vi "test Logging Loopback.vi"(8 "error in":errorcluster, 11 "TestCase in":refnum<class "Logging Loopback.lvclass">) -> (0 "error out":errorcluster, 3 "TestCase out":refnum<class "Logging Loopback.lvclass">)   [LabVIEW 2020, in "Logging Loopback.lvclass"]
uses:
  Logging Loopback.lvclass
  <vilib>/addons/_JKI Toolkits/VI Tester/TestCase.llb/TestCase.lvclass
  <vilib>/NI VeriStand/Execution/Workspace/NI_VS Workspace ExecutionAPI.lvlib
  niveristand-custom-device-testing-tools/VeriStandTestUtilities/VeriStandTestUtilities.lvlib
  <vilib>/NI VeriStand/Execution/Workspace/NI VeriStand - Set Multiple Channel Values.vi
  <vilib>/NI VeriStand/Execution/Workspace/NI VeriStand - Get Multiple Channel Values.vi
  deffbcbf-56d6-44bc-a2e8-818e5af24b3f.vi
  <vilib>/NI VeriStand/Execution/Workspace/NI VeriStand - Get Single Channel Value.vi
  6b2bfa70-eeaf-4af2-80f2-6a86f8a7f598.vi
  <vilib>/NI VeriStand/Execution/Workspace/NI VeriStand - Set Single Channel Value.vi
  8c6fca9a-303d-43f5-9dd5-93be59ae7e12.vi
  8e29fdbb-99f4-44e6-93c0-7b36a3c9813a.vi
  f1b300ac-3edd-4135-92f3-1091e6e89550.vi
  <vilib>/numeric/Random Number (Range) U64.vi
  48c03b12-561d-41cc-966c-8db0e8e8288a.vi
  73f23597-aef4-4ff6-a202-43428571e7d8.vi
  14110b57-2ec4-40ff-8532-aa1d9e607739.vi
  11a182cf-1dad-4243-940f-e832a48a190d.vi
  ddb50979-a497-467d-9150-38dd6115816f.vi
  db7b1ca4-f33a-45a5-961e-f51998a9de3e.vi
  C:/dev/niveristand-custom-device-testing-tools/VeriStandTestCase/VeriStandTestCase.lvclass
  C:/Program Files (x86)/National Instruments/LabVIEW 2020/vi.lib/addons/_JKI Toolkits/VI Tester/TestCase.llb/TestCase.lvclass
  C:/dev/niveristand-ballard-milStd1553-custom-device/Source/Custom Device Support/Tests/System/Logging Loopback/Logging Loopback.lvclass
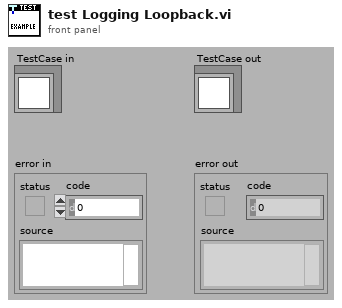
[diagram p1: front panel]
types:
  T1 = typedef "NI_VS Workspace ExecutionAPI.lvlib/WorkspaceAPI.ctl" = refnum<k24>
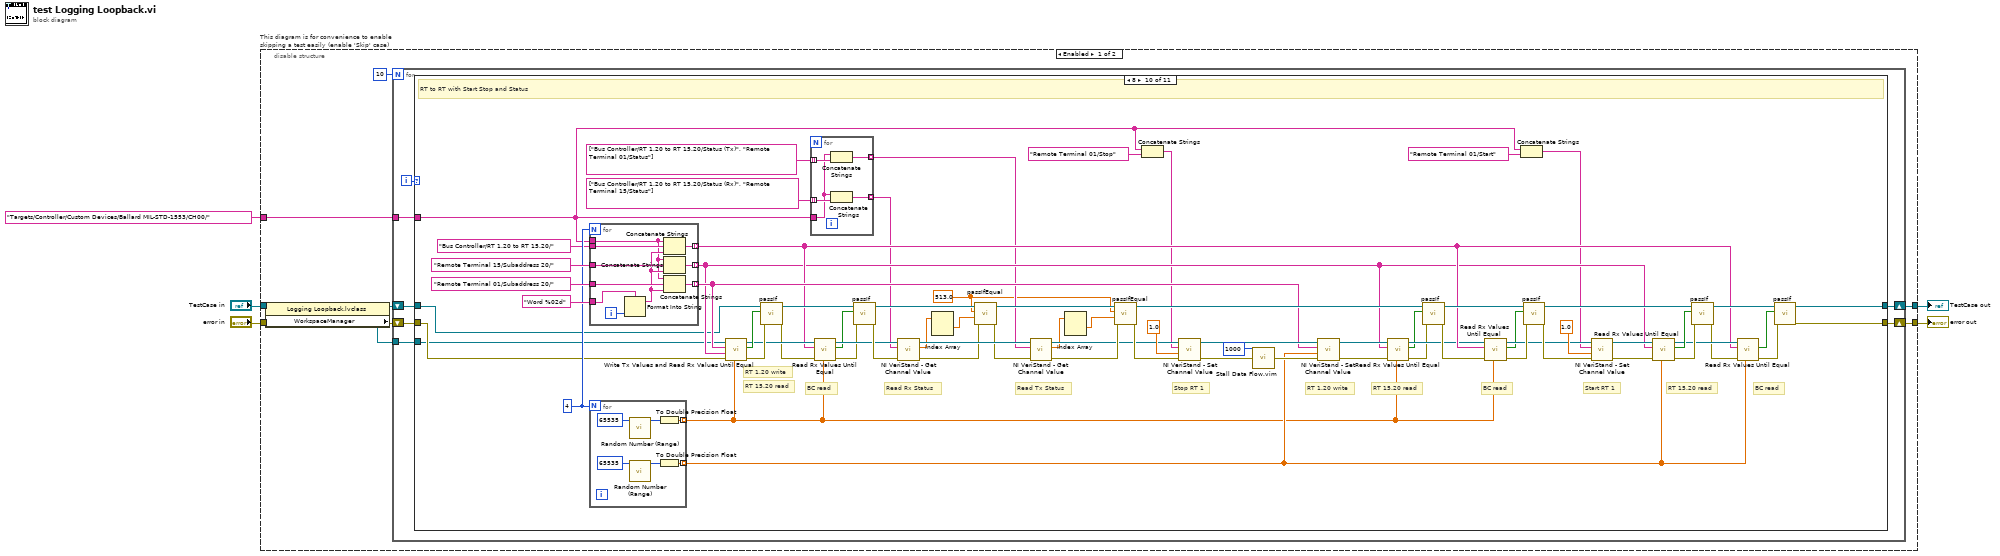
[diagram p0: block diagram]
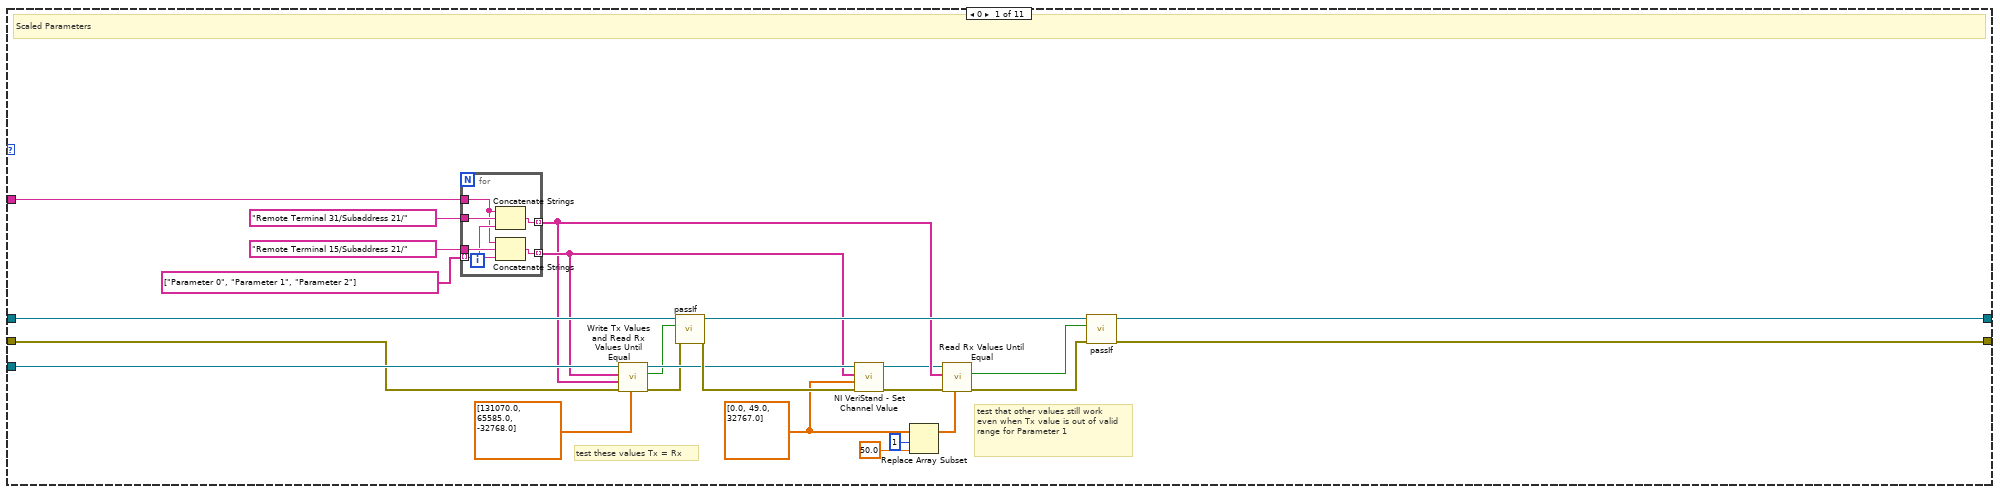
[diagram p2: hidden frame]
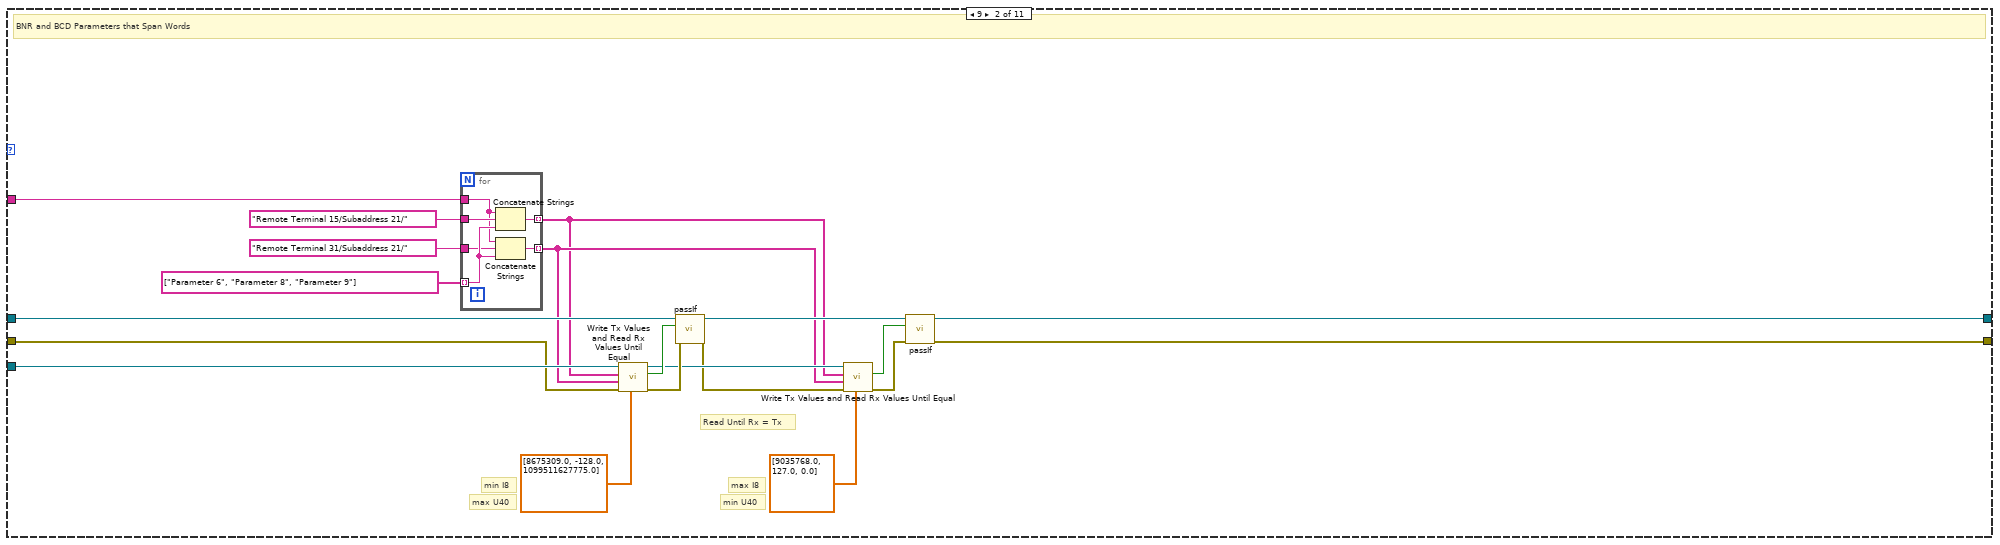
[diagram p3: hidden frame]
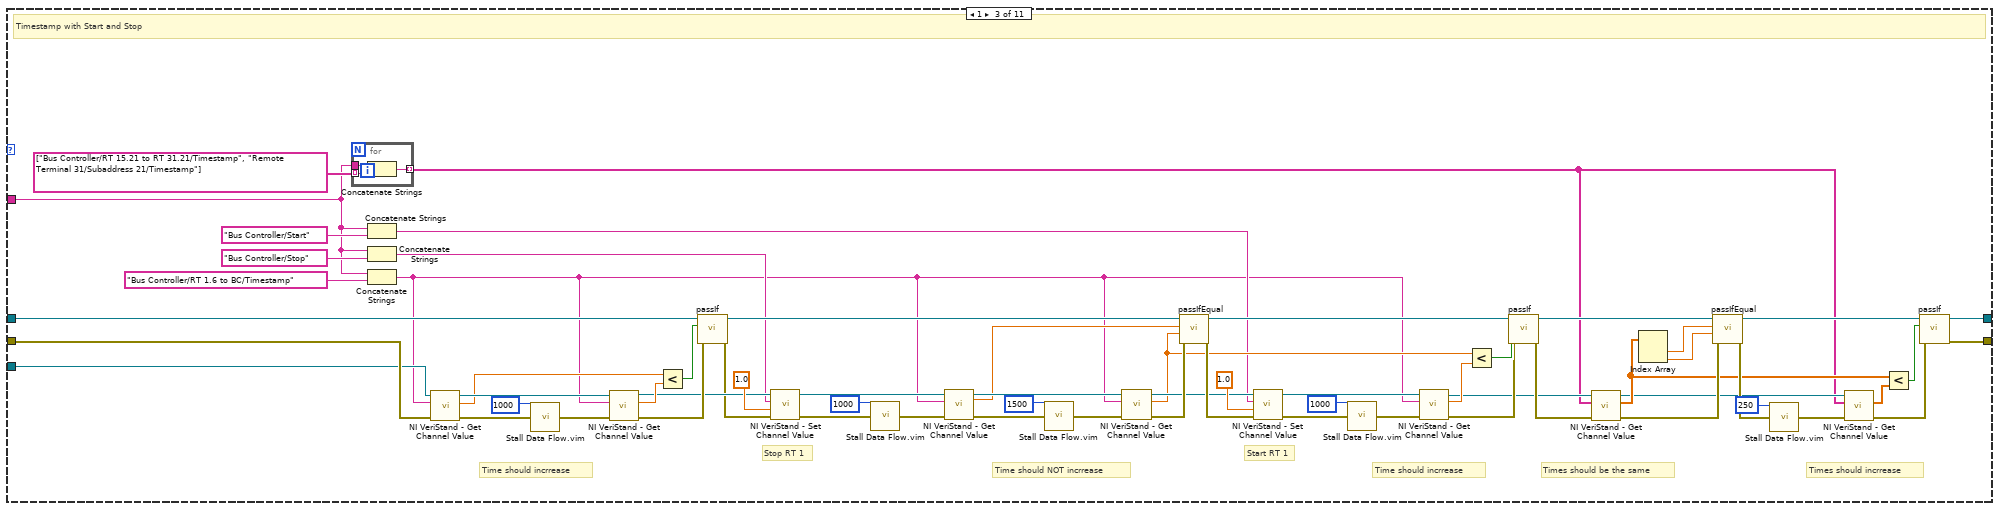
[diagram p4: hidden frame]
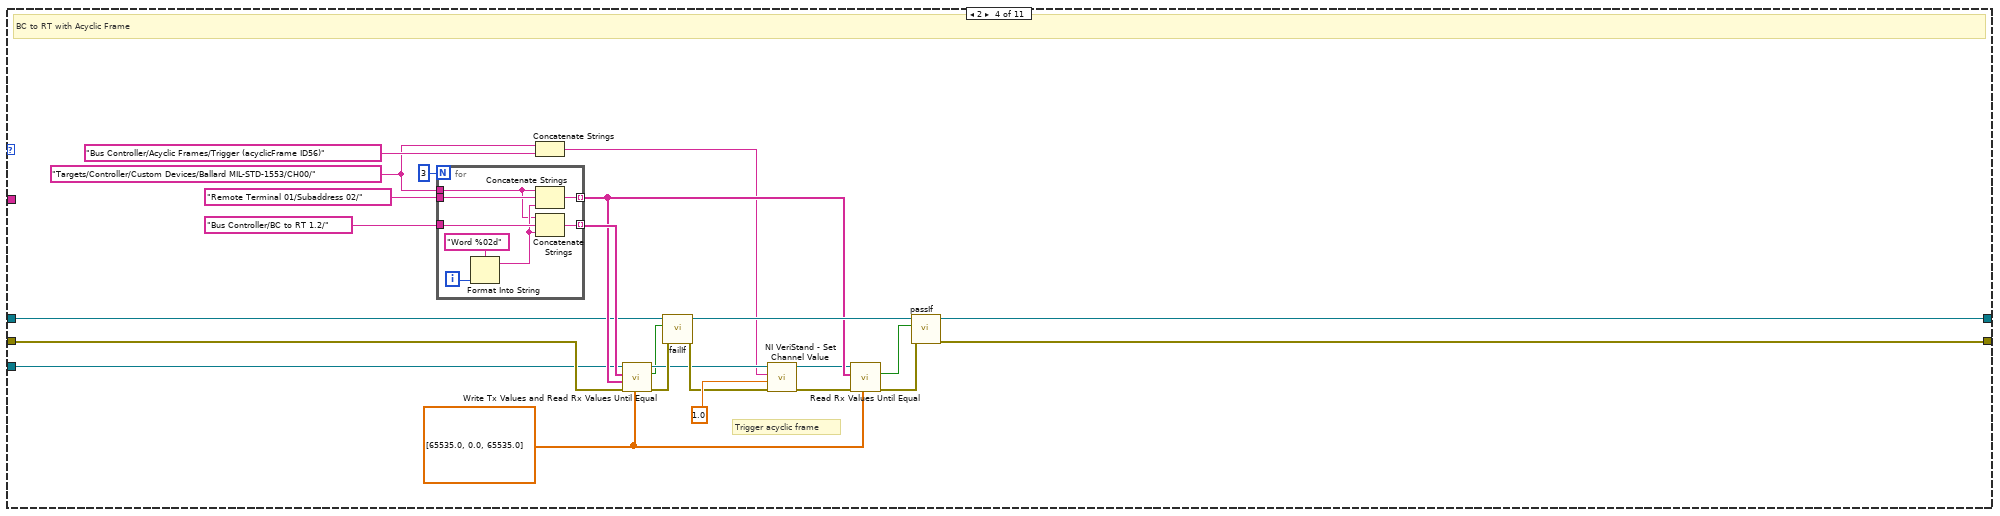
[diagram p5: hidden frame]
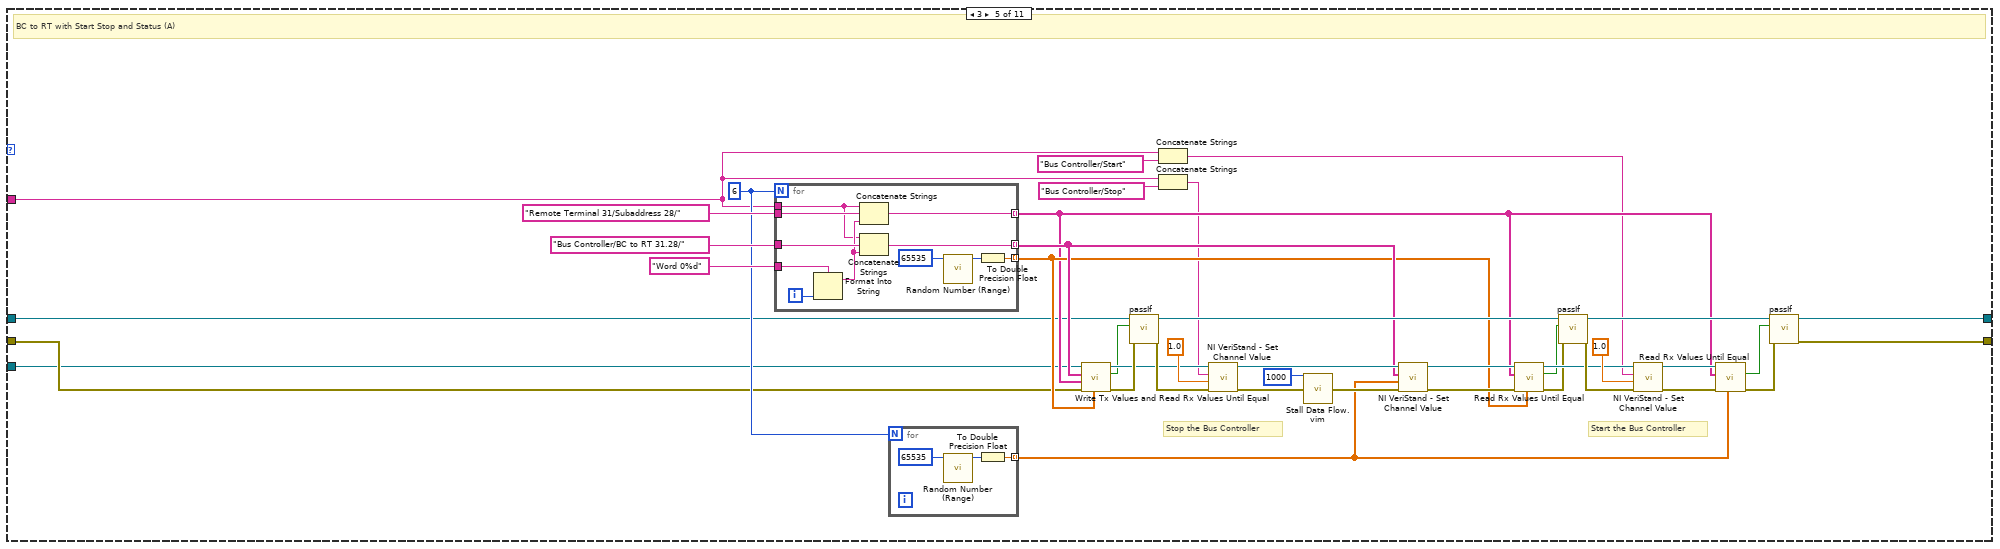
[diagram p6: hidden frame]
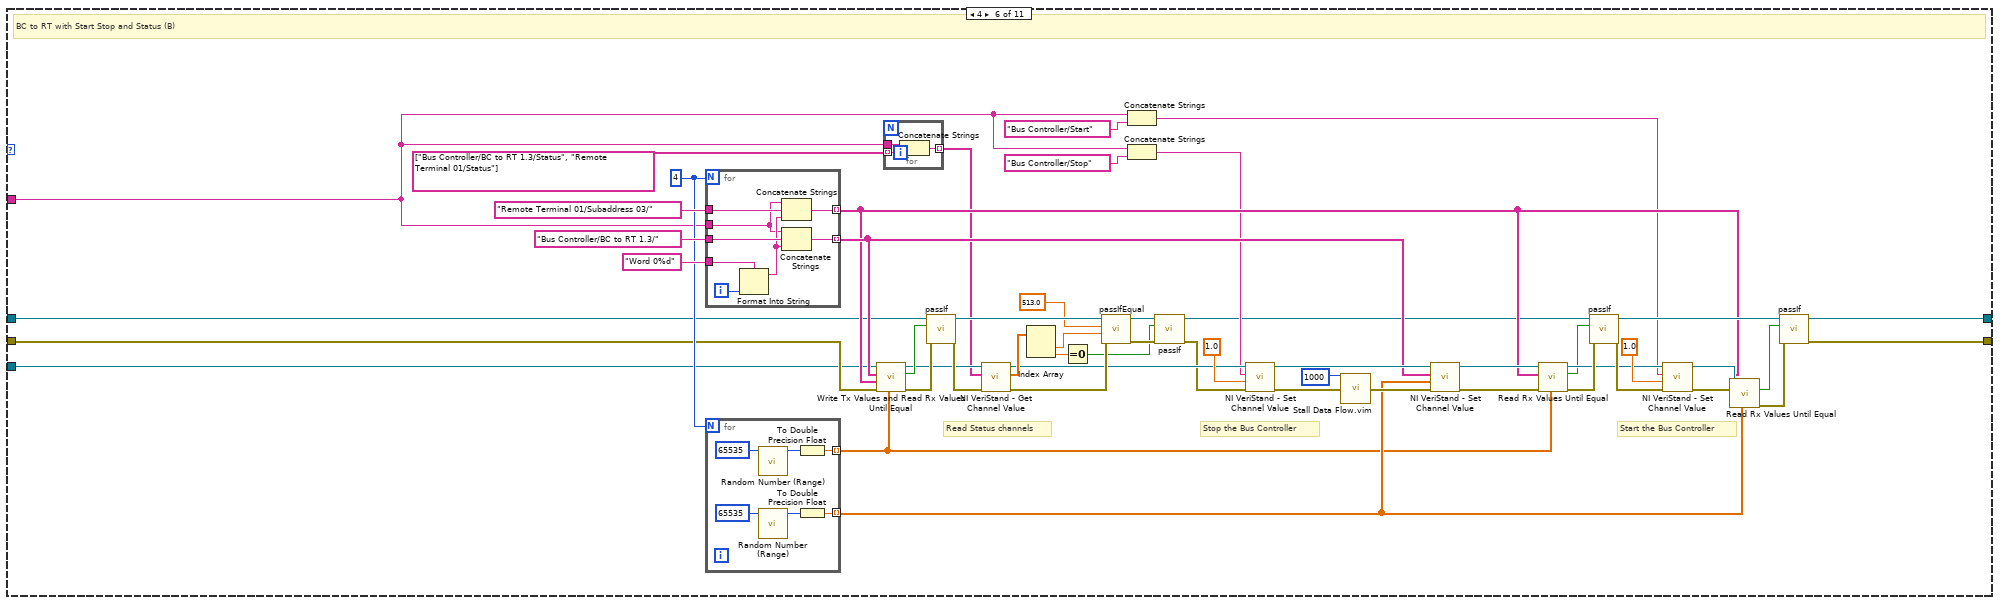
[diagram p7: hidden frame]
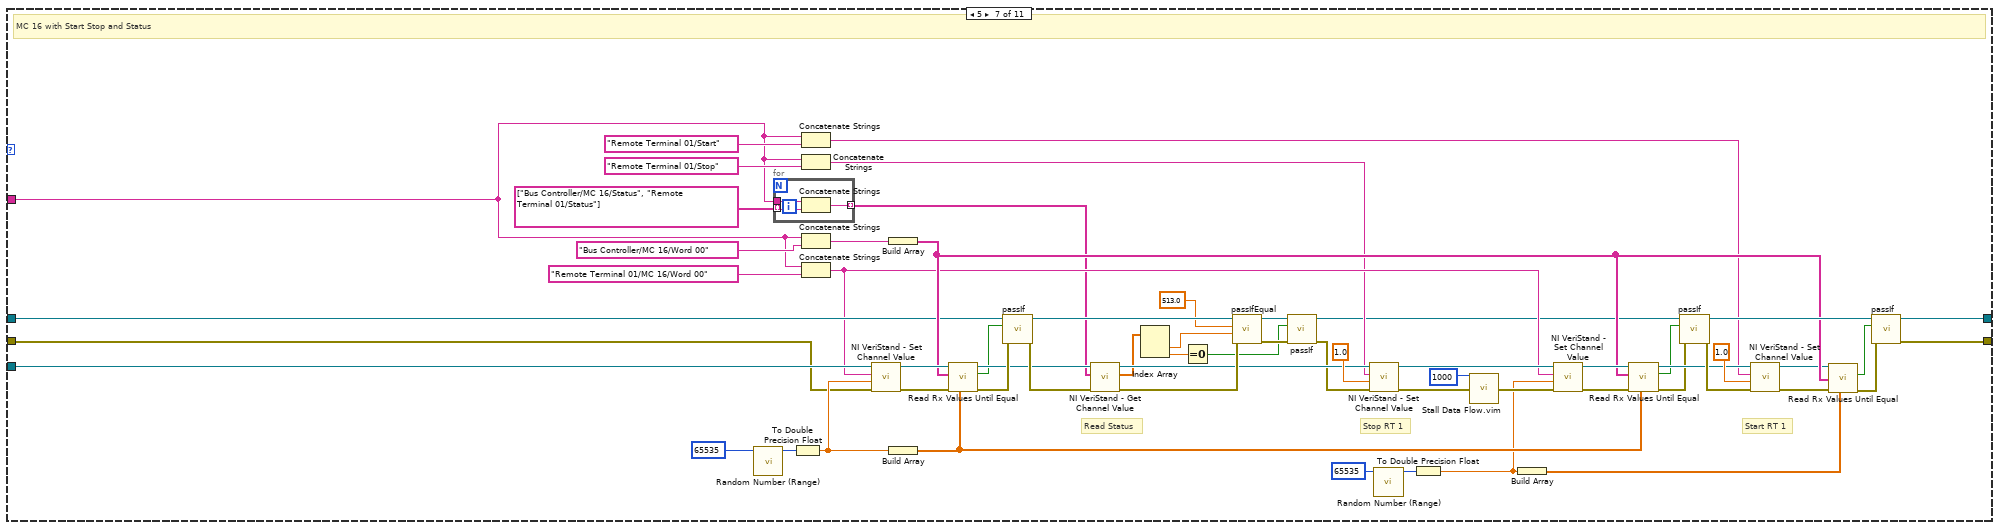
[diagram p8: hidden frame]
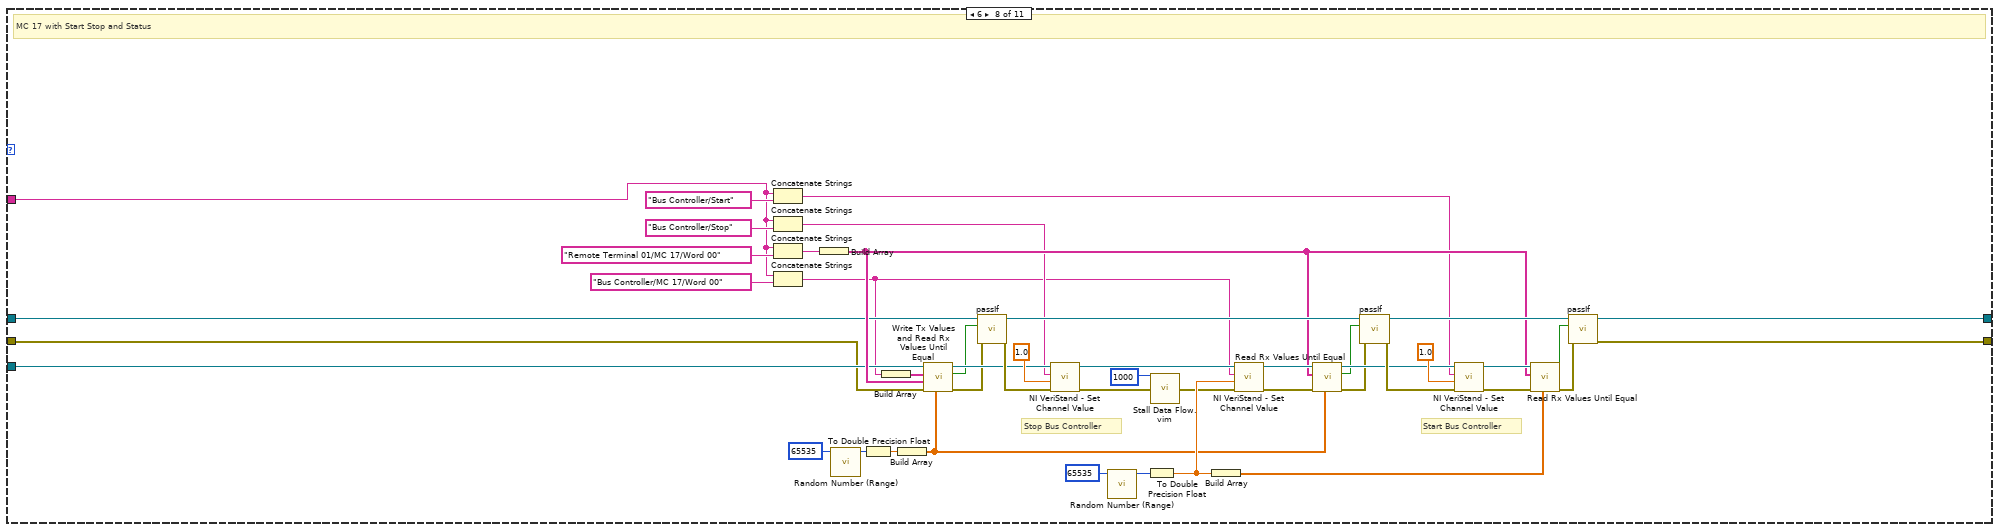
[diagram p9: hidden frame]
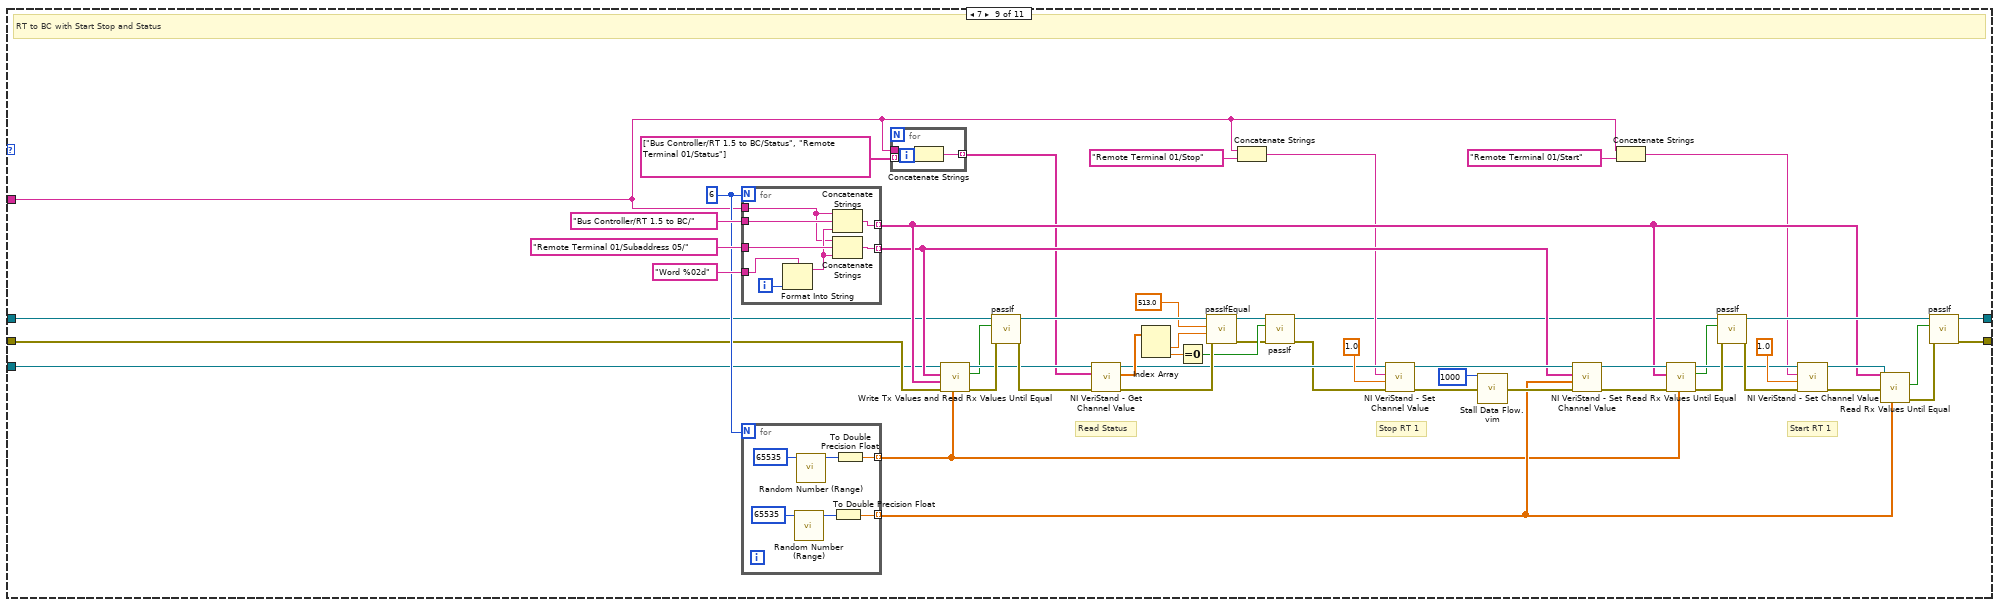
[diagram p10: hidden frame]
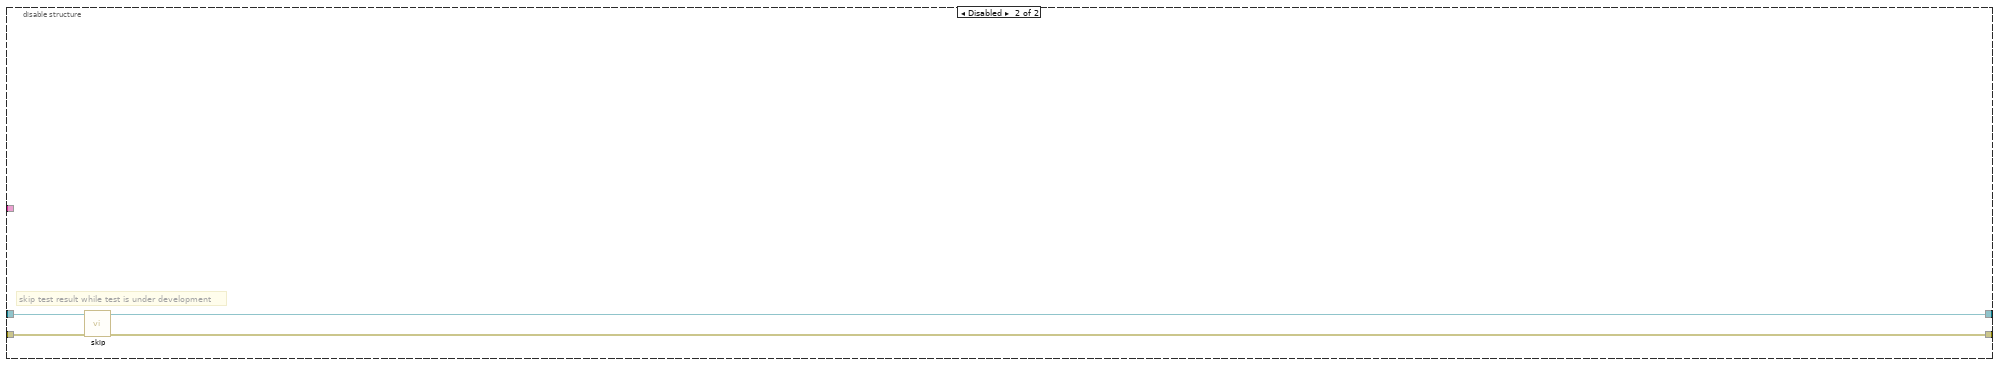
[diagram p12: hidden frame]
diagram:
  n1 = disable-structure "This diagram is for convenience to enable skipping a test easily (enable 'Skip' case)" shown="Enabled" {
    disable-tunnel: "TestCase in" -> [w13 w580]
    disable-tunnel: [w11 w578] -> w2
    disable-tunnel: [w10 w579] -> w4
    disable-tunnel: "error in" -> [w12 w577]
    disable-tunnel: "Targets/Controller/Custom Devices/Ballard MIL-STD-1553/CH00/" ("Channel") -> [w7 _]
    frame Enabled {
      n2 = property class="Logging Loopback.lvclass"(reference=w13, error in=w12) -> (reference out=w14:refnum<class "Logging Loopback.lvclass">, error out=w8:errorcluster, "WorkspaceManager"=w9:T1)
      n3 = for {
        N: 10 -> [_]
        tunnel: w9 -> [w18]
        tunnel: w7 -> [w16]
        shift-right: [w20] -> w11
        shift-left: w14 -> [w21]
        shift-right: [w19] -> w10
        shift-left: w8 -> [w17]
        i -> [w15]
        n4 = case shown="8" w15 {
          tunnel: w21 -> [w46 w72 w85 w149 w177 w243 w323 w375 w429 w483 w576]
          tunnel: [w40 w67 w81 w146 w179 w240 w320 w377 w426 w485 w576] -> w20
          tunnel: [w39 w66 w80 w145 w178 w239 w321 w376 w425 w484 w575] -> w19
          tunnel: w18 -> [w36 w65 w83 w147 w185 w241 w324 w374 w427 w495 _]
          tunnel: w17 -> [w33 w63 w84 w148 w186 w242 w322 w373 w428 w496 w575]
          tunnel: w16 -> [w22 w60 w79 _ w180 w245 w311 w364 w418 w487 _]
          frame 0 {
            w24 = dbl[] [0.0, 49.0, 32767.0] ("appended array")
            # "test that other values still work even when Tx value is out of valid range for Parameter 1"
            # "test these values Tx = Rx"
            # "Scaled Parameters"
            n5 = for {
              tunnel: "Remote Terminal 15/Subaddress 21/" ("Channel") -> [w51]
              tunnel: string[] ["Parameter 0", "Parameter 1", "Parameter 2"] ("Channels") -> [w50] mode=indexing
              tunnel: [w52] -> w31 mode=indexing
              tunnel: "Remote Terminal 31/Subaddress 21/" ("Channel") -> [w49]
              tunnel: [w48] -> w30 mode=indexing
              tunnel: w22 -> [w47]
              n6 = Concatenate Strings(w47, w49, w50) -> (w48:string)
              n7 = Concatenate Strings(w47, w51, w50) -> (w52:string)
            }
            n8 = call "Write Tx Values and Read Rx Values Until Equal.vi"("Tx values"=dbl[] [131070.0, 65585.0, -32768.0] ("appended array"), "error in"=w33, "Rx aliases"=w30, "Tx aliases"=w31, "workspace manager in"=w36) -> ("error out"=w34:errorcluster, "values equal"=w32:bool, "workspace manager out"=w35:T1)  [unwired: 4 in]
            n9 = call-dynamic "passIf.vi"("error in (no error)"=w34, "pass"=w32, "TestCase in"=w46) -> ("error out"=w42:errorcluster, "TestCase out"=w41:refnum<class "Logging Loopback.lvclass">)  [unwired: 7 in]
            n10 = call-poly <vilib>:"NI VeriStand - Set Channel Value.vi"("error in (no error)"=w42, "Values"=w24, "Channels"=w31, "WorkspaceManager in"=w35) -> ("error out"=w29:errorcluster, "WorkspaceManager out"=w28:T1)  [unwired: 6 in]
            n11 = Replace Array Subset(array=w24, new element=50.0 ("x+y"), index=1) -> (w27:dbl[])
            n12 = call "Read Rx Values Until Equal.vi"("expected values"=w27, "error in"=w29, "Rx aliases"=w30, "workspace manager in"=w28) -> ("error out"=w25:errorcluster, "values equal expected"=w26:bool)  [unwired: 5 in, 1 out]
            n13 = call-dynamic "passIf.vi"("error in (no error)"=w25, "pass"=w26, "TestCase in"=w41) -> ("error out"=w39:errorcluster, "TestCase out"=w40:refnum<class "Logging Loopback.lvclass">)  [unwired: 7 in]
          }
          frame 9 {
            # "min U40"
            # "Read Until Rx = Tx"
            # "max I8"
            # "min I8"
            # "max U40"
            # "Read Until Rx = Tx"
            # "BNR and BCD Parameters that Span Words"
            n14 = for {
              tunnel: "Remote Terminal 15/Subaddress 21/" ("Channel") -> [w77]
              tunnel: string[] ["Parameter 6", "Parameter 8", "Parameter 9"] ("Channels") -> [w76] mode=indexing
              tunnel: [w78] -> w56 mode=indexing
              tunnel: "Remote Terminal 31/Subaddress 21/" ("Channel") -> [w75]
              tunnel: [w74] -> w57 mode=indexing
              tunnel: w60 -> [w73]
              n15 = Concatenate Strings(w73, w77, w76) -> (w78:string)
              n16 = Concatenate Strings(w73, w75, w76) -> (w74:string)
            }
            n17 = call "Write Tx Values and Read Rx Values Until Equal.vi"("Tx values"=dbl[] [8675309.0, -128.0, 1099511627775.0] ("appended array"), "error in"=w63, "Rx aliases"=w57, "Tx aliases"=w56, "workspace manager in"=w65) -> ("error out"=w64:errorcluster, "values equal"=w62:bool, "workspace manager out"=w59:T1)  [unwired: 4 in]
            n18 = call-dynamic "passIf.vi"("error in (no error)"=w64, "pass"=w62, "TestCase in"=w72) -> ("error out"=w58:errorcluster, "TestCase out"=w68:refnum<class "Logging Loopback.lvclass">)  [unwired: 7 in]
            n19 = call "Write Tx Values and Read Rx Values Until Equal.vi"("Tx values"=dbl[] [9035768.0, 127.0, 0.0] ("appended array"), "error in"=w58, "Rx aliases"=w57, "Tx aliases"=w56, "workspace manager in"=w59) -> ("error out"=w55:errorcluster, "values equal"=w54:bool)  [unwired: 4 in, 1 out]
            n20 = call-dynamic "passIf.vi"("error in (no error)"=w55, "pass"=w54, "TestCase in"=w68) -> ("error out"=w66:errorcluster, "TestCase out"=w67:refnum<class "Logging Loopback.lvclass">)  [unwired: 7 in]
          }
          frame 1 {
            # "Time should incrrease"
            # "Start RT 1"
            # "Time should NOT incrrease"
            # "Stop RT 1"
            # "Times should incrrease"
            # "Times should be the same"
            # "Time should incrrease"
            # "Timestamp with Start and Stop"
            n21 = for {
              tunnel: string[] ["Bus Controller/RT 15.21 to RT 31.21/Timestamp", "Remote Terminal 31/Subaddress 21/Timestamp"] ("Channels") -> [w144] mode=indexing
              tunnel: w79 -> [w143]
              tunnel: [w142] -> w86 mode=indexing
              n22 = Concatenate Strings(w143, w144) -> (w142:string)
            }
            n23 = Concatenate Strings(w79, "Bus Controller/Start" ("Channel")) -> (w91:string)
            n24 = Concatenate Strings(w79, "Bus Controller/Stop" ("Channel")) -> (w89:string)
            n25 = Concatenate Strings(w79, "Bus Controller/RT 1.6 to BC/Timestamp") -> (w82:string)
            n26 = call-poly <vilib>:"NI VeriStand - Get Channel Value.vi"("error in (no error)"=w84, "Channel"=w82, "WorkspaceManager in"=w83) -> ("error out"=w139:errorcluster, "Value"=w135:dbl, "WorkspaceManager out"=w141:T1)  [unwired: 6 in]
            n27 = call "Stall Data Flow.vim"("value in"=w139, "milliseconds to wait"=u32 1000) -> ("value out"=w140:errorcluster)  [unwired: 1 out]
            n28 = call-poly <vilib>:"NI VeriStand - Get Channel Value.vi"("error in (no error)"=w140, "Channel"=w82, "WorkspaceManager in"=w141) -> ("error out"=w137:errorcluster, "Value"=w134:dbl, "WorkspaceManager out"=w118:T1)  [unwired: 6 in]
            n29 = Less?(x=w135, y=w134) -> (x < y?=w133:bool)
            n30 = call-dynamic "passIf.vi"("error in (no error)"=w137, "pass"=w133, "TestCase in"=w85) -> ("error out"=w117:errorcluster, "TestCase out"=w110:refnum<class "Logging Loopback.lvclass">)  [unwired: 7 in]
            n31 = call-poly <vilib>:"NI VeriStand - Set Channel Value.vi"("error in (no error)"=w117, "Value"=1.0, "Channel"=w89, "WorkspaceManager in"=w118) -> ("error out"=w120:errorcluster, "WorkspaceManager out"=w114:T1)  [unwired: 6 in]
            n32 = call "Stall Data Flow.vim"("value in"=w120, "milliseconds to wait"=u32 1000) -> ("value out"=w113:errorcluster)  [unwired: 1 out]
            n33 = call-poly <vilib>:"NI VeriStand - Get Channel Value.vi"("error in (no error)"=w113, "Channel"=w82, "WorkspaceManager in"=w114) -> ("error out"=w115:errorcluster, "Value"=w109:dbl, "WorkspaceManager out"=w112:T1)  [unwired: 6 in]
            n34 = call "Stall Data Flow.vim"("value in"=w115, "milliseconds to wait"=u32 1500) -> ("value out"=w111:errorcluster)  [unwired: 1 out]
            n35 = call-poly <vilib>:"NI VeriStand - Get Channel Value.vi"("error in (no error)"=w111, "Channel"=w82, "WorkspaceManager in"=w112) -> ("error out"=w108:errorcluster, "Value"=w98:dbl, "WorkspaceManager out"=w102:T1)  [unwired: 6 in]
            n36 = call-dynamic "passIfEqual.vi"("error in (no error)"=w108, "y"=w98, "x"=w109, "TestCase in"=w110) -> ("error out"=w103:errorcluster, "TestCase out"=w97:refnum<class "Logging Loopback.lvclass">)  [unwired: 6 in]
            n37 = call-poly <vilib>:"NI VeriStand - Set Channel Value.vi"("error in (no error)"=w103, "Value"=1.0, "Channel"=w91, "WorkspaceManager in"=w102) -> ("error out"=w105:errorcluster, "WorkspaceManager out"=w107:T1)  [unwired: 6 in]
            n38 = call "Stall Data Flow.vim"("value in"=w105, "milliseconds to wait"=u32 1000) -> ("value out"=w101:errorcluster)  [unwired: 1 out]
            n39 = call-poly <vilib>:"NI VeriStand - Get Channel Value.vi"("error in (no error)"=w101, "Channel"=w82, "WorkspaceManager in"=w107) -> ("error out"=w96:errorcluster, "Value"=w99:dbl, "WorkspaceManager out"=w94:T1)  [unwired: 6 in]
            n40 = Less?(x=w98, y=w99) -> (x < y?=w100:bool)
            n41 = call-dynamic "passIf.vi"("error in (no error)"=w96, "pass"=w100, "TestCase in"=w97) -> ("error out"=w95:errorcluster, "TestCase out"=w93:refnum<class "Logging Loopback.lvclass">)  [unwired: 7 in]
            n42 = call-poly <vilib>:"NI VeriStand - Get Channel Value.vi"("error in (no error)"=w95, "Channels"=w86, "WorkspaceManager in"=w94) -> ("error out"=w136:errorcluster, "Values"=w125:dbl[], "WorkspaceManager out"=w123:T1)  [unwired: 6 in]
            n43 = Index Array(array=w125) -> (element #1=w132:dbl, element #2=w131:dbl)  [unwired: 2 in]
            n44 = call-dynamic "passIfEqual.vi"("error in (no error)"=w136, "y"=w131, "x"=w132, "TestCase in"=w93) -> ("error out"=w130:errorcluster, "TestCase out"=w122:refnum<class "Logging Loopback.lvclass">)  [unwired: 6 in]
            n45 = call "Stall Data Flow.vim"("value in"=w130, "milliseconds to wait"=u32 250) -> ("value out"=w128:errorcluster)  [unwired: 1 out]
            n46 = call-poly <vilib>:"NI VeriStand - Get Channel Value.vi"("error in (no error)"=w128, "Channels"=w86, "WorkspaceManager in"=w123) -> ("error out"=w126:errorcluster, "Values"=w124:dbl[])  [unwired: 6 in, 1 out]
            n47 = Less?(x=w125, y=w124) -> (x < y?=w127:bool)
            n48 = call-dynamic "passIf.vi"("error in (no error)"=w126, "pass"=w127, "TestCase in"=w122) -> ("error out"=w80:errorcluster, "TestCase out"=w81:refnum<class "Logging Loopback.lvclass">)  [unwired: 7 in]
          }
          frame 2 {
            w151 = "Targets/Controller/Custom Devices/Ballard MIL-STD-1553/CH00/" ("Channel")
            w153 = dbl[] [65535.0, 0.0, 65535.0]
            # "Trigger acyclic frame"
            # "BC to RT with Acyclic Frame"
            n49 = for {
              N: 3 -> [_]
              tunnel: "Bus Controller/BC to RT 1.2/" ("Channel") -> [w175]
              tunnel: [w176] -> w162 mode=indexing
              tunnel: "Remote Terminal 01/Subaddress 02/" ("Channel") -> [w174]
              tunnel: [w173] -> w160 mode=indexing
              tunnel: w151 -> [w169]
              i -> [w172]
              n50 = Format Into String(format string="Word %02d", w172) -> (resulting string=w171:string)  [unwired: 2 in, 1 out]
              n51 = Concatenate Strings(w169, w174, w171) -> (w173:string)
              n52 = Concatenate Strings(w169, w175, w171) -> (w176:string)
            }
            n53 = Concatenate Strings(w151, "Bus Controller/Acyclic Frames/Trigger (acyclicFrame ID56)") -> (w150:string)
            n54 = call "Write Tx Values and Read Rx Values Until Equal.vi"("Tx values"=w153, "error in"=w148, "Rx aliases"=w160, "Tx aliases"=w162, "workspace manager in"=w147) -> ("error out"=w161:errorcluster, "values equal"=w154:bool, "workspace manager out"=w158:T1)  [unwired: 4 in]
            n55 = call-dynamic "failIf.vi"("error in (no error)"=w161, "fail"=w154, "TestCase in"=w149) -> ("error out"=w164:errorcluster, "TestCase out"=w163:refnum<class "Logging Loopback.lvclass">)  [unwired: 7 in]
            n56 = call-poly <vilib>:"NI VeriStand - Set Channel Value.vi"("error in (no error)"=w164, "Value"=1.0, "Channel"=w150, "WorkspaceManager in"=w158) -> ("error out"=w155:errorcluster, "WorkspaceManager out"=w156:T1)  [unwired: 6 in]
            n57 = call "Read Rx Values Until Equal.vi"("expected values"=w153, "error in"=w155, "Rx aliases"=w160, "workspace manager in"=w156) -> ("error out"=w157:errorcluster, "values equal expected"=w159:bool)  [unwired: 5 in, 1 out]
            n58 = call-dynamic "passIf.vi"("error in (no error)"=w157, "pass"=w159, "TestCase in"=w163) -> ("error out"=w145:errorcluster, "TestCase out"=w146:refnum<class "Logging Loopback.lvclass">)  [unwired: 7 in]
          }
          frame 3 {
            w202 = 6
            # "Start the Bus Controller"
            # "Stop the Bus Controller"
            # "BC to RT with Start Stop and Status (A)"
            n59 = for {
              N: w202 -> [_]
              tunnel: "Bus Controller/BC to RT 31.28/" ("Channel") -> [w226]
              tunnel: [w227] -> w201 mode=indexing
              tunnel: "Remote Terminal 31/Subaddress 28/" ("Channel") -> [w225]
              tunnel: [w224] -> w190 mode=indexing
              tunnel: "Word 0%d" -> [w222]
              tunnel: [w218] -> w195 mode=indexing
              tunnel: w180 -> [w217]
              i -> [w223]
              n60 = Format Into String(format string=w222, w223) -> (resulting string=w221:string)  [unwired: 2 in, 1 out]
              n61 = Concatenate Strings(w217, w225, w221) -> (w224:string)
              n62 = Concatenate Strings(w217, w226, w221) -> (w227:string)
              n63 = call-poly <vilib>:"Random Number (Range).vi"("upper bound (100)"=u64 65535) -> ("number"=w220:u64)  [unwired: 10 in]
              n64 = To Double Precision Float(number=w220) -> (double precision float=w218:dbl)
            }
            n65 = for {
              N: w202 -> [_]
              tunnel: [w228] -> w187 mode=indexing
              n66 = call-poly <vilib>:"Random Number (Range).vi"("upper bound (100)"=u64 65535) -> ("number"=w229:u64)  [unwired: 10 in]
              n67 = To Double Precision Float(number=w229) -> (double precision float=w228:dbl)
            }
            n68 = call "Write Tx Values and Read Rx Values Until Equal.vi"("Tx values"=w195, "error in"=w186, "Rx aliases"=w190, "Tx aliases"=w201, "workspace manager in"=w185) -> ("error out"=w200:errorcluster, "values equal"=w198:bool, "workspace manager out"=w199:T1)  [unwired: 4 in]
            n69 = call-dynamic "passIf.vi"("error in (no error)"=w200, "pass"=w198, "TestCase in"=w177) -> ("error out"=w204:errorcluster, "TestCase out"=w203:refnum<class "Logging Loopback.lvclass">)  [unwired: 7 in]
            n70 = Concatenate Strings(w180, "Bus Controller/Start" ("Channel")) -> (w183:string)
            n71 = Concatenate Strings(w180, "Bus Controller/Stop" ("Channel")) -> (w181:string)
            n72 = call-poly <vilib>:"NI VeriStand - Set Channel Value.vi"("error in (no error)"=w204, "Value"=1.0, "Channel"=w181, "WorkspaceManager in"=w199) -> ("error out"=w212:errorcluster, "WorkspaceManager out"=w206:T1)  [unwired: 6 in]
            n73 = call "Stall Data Flow.vim"("value in"=w212, "milliseconds to wait"=u32 1000) -> ("value out"=w213:errorcluster)  [unwired: 1 out]
            n74 = call-poly <vilib>:"NI VeriStand - Set Channel Value.vi"("error in (no error)"=w213, "Values"=w187, "Channels"=w201, "WorkspaceManager in"=w206) -> ("error out"=w196:errorcluster, "WorkspaceManager out"=w197:T1)  [unwired: 6 in]
            n75 = call "Read Rx Values Until Equal.vi"("expected values"=w195, "error in"=w196, "Rx aliases"=w190, "workspace manager in"=w197) -> ("error out"=w193:errorcluster, "values equal expected"=w192:bool, "workspace manager out"=w194:T1)  [unwired: 5 in]
            n76 = call-dynamic "passIf.vi"("error in (no error)"=w193, "pass"=w192, "TestCase in"=w203) -> ("error out"=w209:errorcluster, "TestCase out"=w210:refnum<class "Logging Loopback.lvclass">)  [unwired: 7 in]
            n77 = call-poly <vilib>:"NI VeriStand - Set Channel Value.vi"("error in (no error)"=w209, "Value"=1.0, "Channel"=w183, "WorkspaceManager in"=w194) -> ("error out"=w208:errorcluster, "WorkspaceManager out"=w191:T1)  [unwired: 6 in]
            n78 = call "Read Rx Values Until Equal.vi"("expected values"=w187, "error in"=w208, "Rx aliases"=w190, "workspace manager in"=w191) -> ("error out"=w188:errorcluster, "values equal expected"=w189:bool)  [unwired: 5 in, 1 out]
            n79 = call-dynamic "passIf.vi"("error in (no error)"=w188, "pass"=w189, "TestCase in"=w210) -> ("error out"=w178:errorcluster, "TestCase out"=w179:refnum<class "Logging Loopback.lvclass">)  [unwired: 7 in]
          }
          frame 4 {
            w272 = 4
            # "Read Status channels"
            # "Start the Bus Controller"
            # "Stop the Bus Controller"
            # "BC to RT with Start Stop and Status (B)"
            n80 = for {
              N: w272 -> [_]
              tunnel: "Bus Controller/BC to RT 1.3/" ("Channel") -> [w293]
              tunnel: [w294] -> w266 mode=indexing
              tunnel: "Remote Terminal 01/Subaddress 03/" ("Channel") -> [w292]
              tunnel: [w291] -> w255 mode=indexing
              tunnel: "Word 0%d" -> [w289]
              tunnel: w245 -> [w287]
              i -> [w290]
              n81 = Format Into String(format string=w289, w290) -> (resulting string=w288:string)  [unwired: 2 in, 1 out]
              n82 = Concatenate Strings(w287, w292, w288) -> (w291:string)
              n83 = Concatenate Strings(w287, w293, w288) -> (w294:string)
            }
            n84 = for {
              N: w272 -> [_]
              tunnel: [w298] -> w254 mode=indexing
              tunnel: [w295] -> w244 mode=indexing
              n85 = call-poly <vilib>:"Random Number (Range).vi"("upper bound (100)"=u64 65535) -> ("number"=w297:u64)  [unwired: 10 in]
              n86 = call-poly <vilib>:"Random Number (Range).vi"("upper bound (100)"=u64 65535) -> ("number"=w299:u64)  [unwired: 10 in]
              n87 = To Double Precision Float(number=w297) -> (double precision float=w295:dbl)
              n88 = To Double Precision Float(number=w299) -> (double precision float=w298:dbl)
            }
            n89 = call "Write Tx Values and Read Rx Values Until Equal.vi"("Tx values"=w244, "error in"=w242, "Rx aliases"=w255, "Tx aliases"=w266, "workspace manager in"=w241) -> ("error out"=w265:errorcluster, "values equal"=w264:bool, "workspace manager out"=w263:T1)  [unwired: 4 in]
            n90 = for {
              tunnel: string[] ["Bus Controller/BC to RT 1.3/Status", "Remote Terminal 01/Status"] -> [w286] mode=indexing
              tunnel: [w285] -> w246 mode=indexing
              tunnel: w245 -> [w284]
              n91 = Concatenate Strings(w284, w286) -> (w285:string)
            }
            n92 = call-dynamic "passIf.vi"("error in (no error)"=w265, "pass"=w264, "TestCase in"=w243) -> ("error out"=w270:errorcluster, "TestCase out"=w269:refnum<class "Logging Loopback.lvclass">)  [unwired: 7 in]
            n93 = call-poly <vilib>:"NI VeriStand - Get Channel Value.vi"("error in (no error)"=w270, "Channels"=w246, "WorkspaceManager in"=w263) -> ("error out"=w271:errorcluster, "Values"=w268:dbl[], "WorkspaceManager out"=w267:T1)  [unwired: 6 in]
            n94 = Index Array(array=w268) -> (element #1=w238:dbl, element #2=w231:dbl)  [unwired: 2 in]
            n95 = Equal To 0?(x=w231) -> (x = 0?=w232:bool)
            n96 = call-dynamic "passIfEqual.vi"("error in (no error)"=w271, "y"=w238, "x"=513.0 ("element"), "TestCase in"=w269) -> ("error out"=w235:errorcluster, "TestCase out"=w236:refnum<class "Logging Loopback.lvclass">)  [unwired: 6 in]
            n97 = Concatenate Strings(w245, "Bus Controller/Start" ("Channel")) -> (w248:string)
            n98 = Concatenate Strings(w245, "Bus Controller/Stop" ("Channel")) -> (w250:string)
            n99 = call-dynamic "passIf.vi"("error in (no error)"=w235, "pass"=w232, "TestCase in"=w236) -> ("error out"=w234:errorcluster, "TestCase out"=w233:refnum<class "Logging Loopback.lvclass">)  [unwired: 7 in]
            n100 = call-poly <vilib>:"NI VeriStand - Set Channel Value.vi"("error in (no error)"=w234, "Value"=1.0, "Channel"=w250, "WorkspaceManager in"=w267) -> ("error out"=w274:errorcluster, "WorkspaceManager out"=w279:T1)  [unwired: 6 in]
            n101 = call "Stall Data Flow.vim"("value in"=w274, "milliseconds to wait"=u32 1000) -> ("value out"=w273:errorcluster)  [unwired: 1 out]
            n102 = call-poly <vilib>:"NI VeriStand - Set Channel Value.vi"("error in (no error)"=w273, "Values"=w254, "Channels"=w266, "WorkspaceManager in"=w279) -> ("error out"=w261:errorcluster, "WorkspaceManager out"=w262:T1)  [unwired: 6 in]
            n103 = call "Read Rx Values Until Equal.vi"("expected values"=w244, "error in"=w261, "Rx aliases"=w255, "workspace manager in"=w262) -> ("error out"=w260:errorcluster, "values equal expected"=w258:bool, "workspace manager out"=w259:T1)  [unwired: 5 in]
            n104 = call-dynamic "passIf.vi"("error in (no error)"=w260, "pass"=w258, "TestCase in"=w233) -> ("error out"=w277:errorcluster, "TestCase out"=w276:refnum<class "Logging Loopback.lvclass">)  [unwired: 7 in]
            n105 = call-poly <vilib>:"NI VeriStand - Set Channel Value.vi"("error in (no error)"=w277, "Value"=1.0, "Channel"=w248, "WorkspaceManager in"=w259) -> ("error out"=w256:errorcluster, "WorkspaceManager out"=w257:T1)  [unwired: 6 in]
            n106 = call "Read Rx Values Until Equal.vi"("expected values"=w254, "error in"=w256, "Rx aliases"=w255, "workspace manager in"=w257) -> ("error out"=w253:errorcluster, "values equal expected"=w252:bool)  [unwired: 5 in, 1 out]
            n107 = call-dynamic "passIf.vi"("error in (no error)"=w253, "pass"=w252, "TestCase in"=w276) -> ("error out"=w239:errorcluster, "TestCase out"=w240:refnum<class "Logging Loopback.lvclass">)  [unwired: 7 in]
          }
          frame 5 {
            # "Read Status"
            # "Start RT 1"
            # "Stop RT 1"
            # "MC 16 with Start Stop and Status"
            n108 = call-poly <vilib>:"Random Number (Range).vi"("upper bound (100)"=u64 65535) -> ("number"=w360:u64)  [unwired: 10 in]
            n109 = for {
              tunnel: string[] ["Bus Controller/MC 16/Status", "Remote Terminal 01/Status"] -> [w363] mode=indexing
              tunnel: w311 -> [w362]
              tunnel: [w361] -> w309 mode=indexing
              n110 = Concatenate Strings(w362, w363) -> (w361:string)
            }
            n111 = To Double Precision Float(number=w360) -> (double precision float=w343:dbl)
            n112 = Concatenate Strings(w311, "Remote Terminal 01/Start" ("Channel")) -> (w314:string)
            n113 = Concatenate Strings(w311, "Remote Terminal 01/Stop" ("Channel")) -> (w312:string)
            n114 = Concatenate Strings(w311, "Bus Controller/MC 16/Word 00" ("Channel")) -> (w318:string)
            n115 = Concatenate Strings(w311, "Remote Terminal 01/MC 16/Word 00" ("Channel")) -> (w316:string)
            n116 = call-poly <vilib>:"NI VeriStand - Set Channel Value.vi"("error in (no error)"=w322, "Value"=w343, "Channel"=w316, "WorkspaceManager in"=w324) -> ("error out"=w341:errorcluster, "WorkspaceManager out"=w342:T1)  [unwired: 6 in]
            n117 = Build Array(w318) -> (w331:string[])
            n118 = Build Array(w343) -> (w335:dbl[])
            n119 = call "Read Rx Values Until Equal.vi"("expected values"=w335, "error in"=w341, "Rx aliases"=w331, "workspace manager in"=w342) -> ("error out"=w340:errorcluster, "values equal expected"=w338:bool, "workspace manager out"=w339:T1)  [unwired: 5 in]
            n120 = call-dynamic "passIf.vi"("error in (no error)"=w340, "pass"=w338, "TestCase in"=w323) -> ("error out"=w347:errorcluster, "TestCase out"=w346:refnum<class "Logging Loopback.lvclass">)  [unwired: 7 in]
            n121 = call-poly <vilib>:"NI VeriStand - Get Channel Value.vi"("error in (no error)"=w347, "Channels"=w309, "WorkspaceManager in"=w339) -> ("error out"=w348:errorcluster, "Values"=w344:dbl[], "WorkspaceManager out"=w345:T1)  [unwired: 6 in]
            n122 = Index Array(array=w344) -> (element #1=w307:dbl, element #2=w308:dbl)  [unwired: 2 in]
            n123 = Equal To 0?(x=w308) -> (x = 0?=w302:bool)
            n124 = call-dynamic "passIfEqual.vi"("error in (no error)"=w348, "y"=w307, "x"=513.0 ("element"), "TestCase in"=w346) -> ("error out"=w306:errorcluster, "TestCase out"=w304:refnum<class "Logging Loopback.lvclass">)  [unwired: 6 in]
            n125 = call-dynamic "passIf.vi"("error in (no error)"=w306, "pass"=w302, "TestCase in"=w304) -> ("error out"=w305:errorcluster, "TestCase out"=w303:refnum<class "Logging Loopback.lvclass">)  [unwired: 7 in]
            n126 = call-poly <vilib>:"NI VeriStand - Set Channel Value.vi"("error in (no error)"=w305, "Value"=1.0, "Channel"=w312, "WorkspaceManager in"=w345) -> ("error out"=w357:errorcluster, "WorkspaceManager out"=w354:T1)  [unwired: 6 in]
            n127 = call-poly <vilib>:"Random Number (Range).vi"("upper bound (100)"=u64 65535) -> ("number"=w352:u64)  [unwired: 10 in]
            n128 = To Double Precision Float(number=w352) -> (double precision float=w326:dbl)
            n129 = call "Stall Data Flow.vim"("value in"=w357, "milliseconds to wait"=u32 1000) -> ("value out"=w355:errorcluster)  [unwired: 1 out]
            n130 = Build Array(w326) -> (w328:dbl[])
            n131 = call-poly <vilib>:"NI VeriStand - Set Channel Value.vi"("error in (no error)"=w355, "Value"=w326, "Channel"=w316, "WorkspaceManager in"=w354) -> ("error out"=w336:errorcluster, "WorkspaceManager out"=w337:T1)  [unwired: 6 in]
            n132 = call "Read Rx Values Until Equal.vi"("expected values"=w335, "error in"=w336, "Rx aliases"=w331, "workspace manager in"=w337) -> ("error out"=w333:errorcluster, "values equal expected"=w332:bool, "workspace manager out"=w334:T1)  [unwired: 5 in]
            n133 = call-dynamic "passIf.vi"("error in (no error)"=w333, "pass"=w332, "TestCase in"=w303) -> ("error out"=w350:errorcluster, "TestCase out"=w349:refnum<class "Logging Loopback.lvclass">)  [unwired: 7 in]
            n134 = call-poly <vilib>:"NI VeriStand - Set Channel Value.vi"("error in (no error)"=w350, "Value"=1.0, "Channel"=w314, "WorkspaceManager in"=w334) -> ("error out"=w329:errorcluster, "WorkspaceManager out"=w330:T1)  [unwired: 6 in]
            n135 = call "Read Rx Values Until Equal.vi"("expected values"=w328, "error in"=w329, "Rx aliases"=w331, "workspace manager in"=w330) -> ("error out"=w327:errorcluster, "values equal expected"=w325:bool)  [unwired: 5 in, 1 out]
            n136 = call-dynamic "passIf.vi"("error in (no error)"=w327, "pass"=w325, "TestCase in"=w349) -> ("error out"=w321:errorcluster, "TestCase out"=w320:refnum<class "Logging Loopback.lvclass">)  [unwired: 7 in]
          }
          frame 6 {
            # "Start Bus Controller"
            # "Stop Bus Controller"
            # "MC 17 with Start Stop and Status"
            n137 = Concatenate Strings(w364, "Bus Controller/Start" ("Channel")) -> (w371:string)
            n138 = Concatenate Strings(w364, "Bus Controller/Stop" ("Channel")) -> (w369:string)
            n139 = Concatenate Strings(w364, "Remote Terminal 01/MC 17/Word 00" ("Channel")) -> (w367:string)
            n140 = Concatenate Strings(w364, "Bus Controller/MC 17/Word 00" ("Channel")) -> (w365:string)
            n141 = Build Array(w367) -> (w378:string[])
            n142 = call-poly <vilib>:"Random Number (Range).vi"("upper bound (100)"=u64 65535) -> ("number"=w409:u64)  [unwired: 10 in]
            n143 = To Double Precision Float(number=w409) -> (double precision float=w394:dbl)
            n144 = Build Array(w365) -> (w393:string[])
            n145 = Build Array(w394) -> (w385:dbl[])
            n146 = call "Write Tx Values and Read Rx Values Until Equal.vi"("Tx values"=w385, "error in"=w373, "Rx aliases"=w378, "Tx aliases"=w393, "workspace manager in"=w374) -> ("error out"=w391:errorcluster, "values equal"=w390:bool, "workspace manager out"=w392:T1)  [unwired: 4 in]
            n147 = call-dynamic "passIf.vi"("error in (no error)"=w391, "pass"=w390, "TestCase in"=w375) -> ("error out"=w396:errorcluster, "TestCase out"=w395:refnum<class "Logging Loopback.lvclass">)  [unwired: 7 in]
            n148 = call-poly <vilib>:"NI VeriStand - Set Channel Value.vi"("error in (no error)"=w396, "Value"=1.0, "Channel"=w369, "WorkspaceManager in"=w392) -> ("error out"=w398:errorcluster, "WorkspaceManager out"=w401:T1)  [unwired: 6 in]
            n149 = call-poly <vilib>:"Random Number (Range).vi"("upper bound (100)"=u64 65535) -> ("number"=w403:u64)  [unwired: 10 in]
            n150 = To Double Precision Float(number=w403) -> (double precision float=w407:dbl)
            n151 = call "Stall Data Flow.vim"("value in"=w398, "milliseconds to wait"=u32 1000) -> ("value out"=w400:errorcluster)  [unwired: 1 out]
            n152 = Build Array(w407) -> (w381:dbl[])
            n153 = call-poly <vilib>:"NI VeriStand - Set Channel Value.vi"("error in (no error)"=w400, "Value"=w407, "Channel"=w365, "WorkspaceManager in"=w401) -> ("error out"=w388:errorcluster, "WorkspaceManager out"=w389:T1)  [unwired: 6 in]
            n154 = call "Read Rx Values Until Equal.vi"("expected values"=w385, "error in"=w388, "Rx aliases"=w378, "workspace manager in"=w389) -> ("error out"=w386:errorcluster, "values equal expected"=w384:bool, "workspace manager out"=w387:T1)  [unwired: 5 in]
            n155 = call-dynamic "passIf.vi"("error in (no error)"=w386, "pass"=w384, "TestCase in"=w395) -> ("error out"=w405:errorcluster, "TestCase out"=w406:refnum<class "Logging Loopback.lvclass">)  [unwired: 7 in]
            n156 = call-poly <vilib>:"NI VeriStand - Set Channel Value.vi"("error in (no error)"=w405, "Value"=1.0, "Channel"=w371, "WorkspaceManager in"=w387) -> ("error out"=w382:errorcluster, "WorkspaceManager out"=w383:T1)  [unwired: 6 in]
            n157 = call "Read Rx Values Until Equal.vi"("expected values"=w381, "error in"=w382, "Rx aliases"=w378, "workspace manager in"=w383) -> ("error out"=w380:errorcluster, "values equal expected"=w379:bool)  [unwired: 5 in, 1 out]
            n158 = call-dynamic "passIf.vi"("error in (no error)"=w380, "pass"=w379, "TestCase in"=w406) -> ("error out"=w376:errorcluster, "TestCase out"=w377:refnum<class "Logging Loopback.lvclass">)  [unwired: 7 in]
          }
          frame 7 {
            w452 = 6
            # "Read Status"
            # "Start RT 1"
            # "Stop RT 1"
            # "RT to BC with Start Stop and Status"
            n159 = for {
              N: w452 -> [_]
              tunnel: "Remote Terminal 01/Subaddress 05/" ("Channel") -> [w472]
              tunnel: [w473] -> w434 mode=indexing
              tunnel: "Bus Controller/RT 1.5 to BC/" ("Channel") -> [w471]
              tunnel: [w470] -> w435 mode=indexing
              tunnel: "Word %02d" -> [w467]
              tunnel: w418 -> [w466]
              i -> [w469]
              n160 = Format Into String(format string=w467, w469) -> (resulting string=w468:string)  [unwired: 2 in, 1 out]
              n161 = Concatenate Strings(w466, w471, w468) -> (w470:string)
              n162 = Concatenate Strings(w466, w472, w468) -> (w473:string)
            }
            n163 = for {
              N: w452 -> [_]
              tunnel: [w477] -> w443 mode=indexing
              tunnel: [w474] -> w430 mode=indexing
              n164 = call-poly <vilib>:"Random Number (Range).vi"("upper bound (100)"=u64 65535) -> ("number"=w478:u64)  [unwired: 10 in]
              n165 = call-poly <vilib>:"Random Number (Range).vi"("upper bound (100)"=u64 65535) -> ("number"=w476:u64)  [unwired: 10 in]
              n166 = To Double Precision Float(number=w478) -> (double precision float=w477:dbl)
              n167 = To Double Precision Float(number=w476) -> (double precision float=w474:dbl)
            }
            n168 = for {
              tunnel: string[] ["Bus Controller/RT 1.5 to BC/Status", "Remote Terminal 01/Status"] -> [w465] mode=indexing
              tunnel: [w464] -> w423 mode=indexing
              tunnel: w418 -> [w463]
              n169 = Concatenate Strings(w463, w465) -> (w464:string)
            }
            n170 = call "Write Tx Values and Read Rx Values Until Equal.vi"("Tx values"=w430, "error in"=w428, "Rx aliases"=w435, "Tx aliases"=w434, "workspace manager in"=w427) -> ("error out"=w433:errorcluster, "values equal"=w431:bool, "workspace manager out"=w432:T1)  [unwired: 4 in]
            n171 = call-dynamic "passIf.vi"("error in (no error)"=w433, "pass"=w431, "TestCase in"=w429) -> ("error out"=w448:errorcluster, "TestCase out"=w447:refnum<class "Logging Loopback.lvclass">)  [unwired: 7 in]
            n172 = call-poly <vilib>:"NI VeriStand - Get Channel Value.vi"("error in (no error)"=w448, "Channels"=w423, "WorkspaceManager in"=w432) -> ("error out"=w449:errorcluster, "Values"=w450:dbl[], "WorkspaceManager out"=w446:T1)  [unwired: 6 in]
            n173 = Index Array(array=w450) -> (element #1=w417:dbl, element #2=w415:dbl)  [unwired: 2 in]
            n174 = Equal To 0?(x=w415) -> (x = 0?=w414:bool)
            n175 = call-dynamic "passIfEqual.vi"("error in (no error)"=w449, "y"=w417, "x"=513.0 ("element"), "TestCase in"=w447) -> ("error out"=w413:errorcluster, "TestCase out"=w411:refnum<class "Logging Loopback.lvclass">)  [unwired: 6 in]
            n176 = Concatenate Strings(w418, "Remote Terminal 01/Stop" ("Channel")) -> (w421:string)
            n177 = call-dynamic "passIf.vi"("error in (no error)"=w413, "pass"=w414, "TestCase in"=w411) -> ("error out"=w412:errorcluster, "TestCase out"=w410:refnum<class "Logging Loopback.lvclass">)  [unwired: 7 in]
            n178 = call-poly <vilib>:"NI VeriStand - Set Channel Value.vi"("error in (no error)"=w412, "Value"=1.0, "Channel"=w421, "WorkspaceManager in"=w446) -> ("error out"=w454:errorcluster, "WorkspaceManager out"=w458:T1)  [unwired: 6 in]
            n179 = call "Stall Data Flow.vim"("value in"=w454, "milliseconds to wait"=u32 1000) -> ("value out"=w453:errorcluster)  [unwired: 1 out]
            n180 = call-poly <vilib>:"NI VeriStand - Set Channel Value.vi"("error in (no error)"=w453, "Values"=w443, "Channels"=w434, "WorkspaceManager in"=w458) -> ("error out"=w439:errorcluster, "WorkspaceManager out"=w440:T1)  [unwired: 6 in]
            n181 = Concatenate Strings(w418, "Remote Terminal 01/Start" ("Channel")) -> (w419:string)
            n182 = call "Read Rx Values Until Equal.vi"("expected values"=w430, "error in"=w439, "Rx aliases"=w435, "workspace manager in"=w440) -> ("error out"=w438:errorcluster, "values equal expected"=w436:bool, "workspace manager out"=w437:T1)  [unwired: 5 in]
            n183 = call-dynamic "passIf.vi"("error in (no error)"=w438, "pass"=w436, "TestCase in"=w410) -> ("error out"=w456:errorcluster, "TestCase out"=w451:refnum<class "Logging Loopback.lvclass">)  [unwired: 7 in]
            n184 = call-poly <vilib>:"NI VeriStand - Set Channel Value.vi"("error in (no error)"=w456, "Value"=1.0, "Channel"=w419, "WorkspaceManager in"=w437) -> ("error out"=w444:errorcluster, "WorkspaceManager out"=w445:T1)  [unwired: 6 in]
            n185 = call "Read Rx Values Until Equal.vi"("expected values"=w443, "error in"=w444, "Rx aliases"=w435, "workspace manager in"=w445) -> ("error out"=w442:errorcluster, "values equal expected"=w441:bool)  [unwired: 5 in, 1 out]
            n186 = call-dynamic "passIf.vi"("error in (no error)"=w442, "pass"=w441, "TestCase in"=w451) -> ("error out"=w425:errorcluster, "TestCase out"=w426:refnum<class "Logging Loopback.lvclass">)  [unwired: 7 in]
          }
          frame 8 {
            w481 = 513.0 ("element")
            w544 = 4
            # "Read Tx Status"
            # "Read Rx Status"
            # "BC read"
            # "RT 15.20 read"
            # "BC read"
            # "RT 15.20 read"
            # "RT 1.20 write"
            # "BC read"
            # "RT 15.20 read"
            # "RT 1.20 write"
            # "Start RT 1"
            # "Stop RT 1"
            # "RT to RT with Start Stop and Status"
            n187 = for {
              N: w544 -> [_]
              tunnel: "Remote Terminal 01/Subaddress 20/" ("Channel") -> [w567]
              tunnel: [w568] -> w525 mode=indexing
              tunnel: "Remote Terminal 15/Subaddress 20/" ("Channel") -> [w566]
              tunnel: [w565] -> w501 mode=indexing
              tunnel: "Word %02d" -> [w560]
              tunnel: "Bus Controller/RT 1.20 to RT 15.20/" ("Channel") -> [w563]
              tunnel: [w561] -> w508 mode=indexing
              tunnel: w487 -> [w559]
              i -> [w564]
              n188 = Format Into String(format string=w560, w564) -> (resulting string=w562:string)  [unwired: 2 in, 1 out]
              n189 = Concatenate Strings(w559, w563, w562) -> (w561:string)
              n190 = Concatenate Strings(w559, w566, w562) -> (w565:string)
              n191 = Concatenate Strings(w559, w567, w562) -> (w568:string)
            }
            n192 = for {
              N: w544 -> [_]
              tunnel: [w572] -> w510 mode=indexing
              tunnel: [w569] -> w497 mode=indexing
              n193 = call-poly <vilib>:"Random Number (Range).vi"("upper bound (100)"=u64 65535) -> ("number"=w571:u64)  [unwired: 10 in]
              n194 = call-poly <vilib>:"Random Number (Range).vi"("upper bound (100)"=u64 65535) -> ("number"=w573:u64)  [unwired: 10 in]
              n195 = To Double Precision Float(number=w571) -> (double precision float=w569:dbl)
              n196 = To Double Precision Float(number=w573) -> (double precision float=w572:dbl)
            }
            n197 = call "Write Tx Values and Read Rx Values Until Equal.vi"("Tx values"=w497, "error in"=w496, "Rx aliases"=w501, "Tx aliases"=w525, "workspace manager in"=w495) -> ("error out"=w524:errorcluster, "values equal"=w523:bool, "workspace manager out"=w522:T1)  [unwired: 4 in]
            n198 = call-dynamic "passIf.vi"("error in (no error)"=w524, "pass"=w523, "TestCase in"=w483) -> ("error out"=w521:errorcluster, "TestCase out"=w542:refnum<class "Logging Loopback.lvclass">)  [unwired: 7 in]
            n199 = for {
              tunnel: [w558] -> w491 mode=indexing
              tunnel: [w557] -> w492 mode=indexing
              tunnel: string[] ["Bus Controller/RT 1.20 to RT 15.20/Status (Tx)", "Remote Terminal 01/Status"] -> [w556] mode=indexing
              tunnel: string[] ["Bus Controller/RT 1.20 to RT 15.20/Status (Rx)", "Remote Terminal 15/Status"] -> [w555] mode=indexing
              tunnel: w487 -> [w554]
              n200 = Concatenate Strings(w554, w556) -> (w557:string)
              n201 = Concatenate Strings(w554, w555) -> (w558:string)
            }
            n202 = call "Read Rx Values Until Equal.vi"("expected values"=w497, "error in"=w521, "Rx aliases"=w508, "workspace manager in"=w522) -> ("error out"=w519:errorcluster, "values equal expected"=w518:bool, "workspace manager out"=w520:T1)  [unwired: 5 in]
            n203 = call-dynamic "passIf.vi"("error in (no error)"=w519, "pass"=w518, "TestCase in"=w542) -> ("error out"=w532:errorcluster, "TestCase out"=w531:refnum<class "Logging Loopback.lvclass">)  [unwired: 7 in]
            n204 = call-poly <vilib>:"NI VeriStand - Get Channel Value.vi"("error in (no error)"=w532, "Channels"=w491, "WorkspaceManager in"=w520) -> ("error out"=w533:errorcluster, "Values"=w526:dbl[], "WorkspaceManager out"=w537:T1)  [unwired: 6 in]
            n205 = Index Array(array=w526) -> (element #1=w482:dbl)  [unwired: 2 in, 1 out]
            n206 = call-dynamic "passIfEqual.vi"("error in (no error)"=w533, "y"=w482, "x"=w481, "TestCase in"=w531) -> ("error out"=w535:errorcluster, "TestCase out"=w536:refnum<class "Logging Loopback.lvclass">)  [unwired: 6 in]
            n207 = call-poly <vilib>:"NI VeriStand - Get Channel Value.vi"("error in (no error)"=w535, "Channels"=w492, "WorkspaceManager in"=w537) -> ("error out"=w534:errorcluster, "Values"=w527:dbl[], "WorkspaceManager out"=w529:T1)  [unwired: 6 in]
            n208 = Index Array(array=w527) -> (element #1=w480:dbl)  [unwired: 2 in, 1 out]
            n209 = call-dynamic "passIfEqual.vi"("error in (no error)"=w534, "y"=w480, "x"=w481, "TestCase in"=w536) -> ("error out"=w530:errorcluster, "TestCase out"=w528:refnum<class "Logging Loopback.lvclass">)  [unwired: 6 in]
            n210 = Concatenate Strings(w487, "Remote Terminal 01/Stop" ("Channel")) -> (w489:string)
            n211 = call-poly <vilib>:"NI VeriStand - Set Channel Value.vi"("error in (no error)"=w530, "Value"=1.0, "Channel"=w489, "WorkspaceManager in"=w529) -> ("error out"=w546:errorcluster, "WorkspaceManager out"=w549:T1)  [unwired: 6 in]
            n212 = call "Stall Data Flow.vim"("value in"=w546, "milliseconds to wait"=u32 1000) -> ("value out"=w545:errorcluster)  [unwired: 1 out]
            n213 = call-poly <vilib>:"NI VeriStand - Set Channel Value.vi"("error in (no error)"=w545, "Values"=w510, "Channels"=w525, "WorkspaceManager in"=w549) -> ("error out"=w502:errorcluster, "WorkspaceManager out"=w503:T1)  [unwired: 6 in]
            n214 = call "Read Rx Values Until Equal.vi"("expected values"=w497, "error in"=w502, "Rx aliases"=w501, "workspace manager in"=w503) -> ("error out"=w499:errorcluster, "values equal expected"=w498:bool, "workspace manager out"=w500:T1)  [unwired: 5 in]
            n215 = call-dynamic "passIf.vi"("error in (no error)"=w499, "pass"=w498, "TestCase in"=w528) -> ("error out"=w507:errorcluster, "TestCase out"=w539:refnum<class "Logging Loopback.lvclass">)  [unwired: 7 in]
            n216 = call "Read Rx Values Until Equal.vi"("expected values"=w497, "error in"=w507, "Rx aliases"=w508, "workspace manager in"=w500) -> ("error out"=w506:errorcluster, "values equal expected"=w504:bool, "workspace manager out"=w505:T1)  [unwired: 5 in]
            n217 = Concatenate Strings(w487, "Remote Terminal 01/Start" ("Channel")) -> (w486:string)
            n218 = call-dynamic "passIf.vi"("error in (no error)"=w506, "pass"=w504, "TestCase in"=w539) -> ("error out"=w540:errorcluster, "TestCase out"=w538:refnum<class "Logging Loopback.lvclass">)  [unwired: 7 in]
            n219 = call-poly <vilib>:"NI VeriStand - Set Channel Value.vi"("error in (no error)"=w540, "Value"=1.0, "Channel"=w486, "WorkspaceManager in"=w505) -> ("error out"=w516:errorcluster, "WorkspaceManager out"=w517:T1)  [unwired: 6 in]
            n220 = call "Read Rx Values Until Equal.vi"("expected values"=w510, "error in"=w516, "Rx aliases"=w501, "workspace manager in"=w517) -> ("error out"=w514:errorcluster, "values equal expected"=w515:bool, "workspace manager out"=w513:T1)  [unwired: 5 in]
            n221 = call-dynamic "passIf.vi"("error in (no error)"=w514, "pass"=w515, "TestCase in"=w538) -> ("error out"=w512:errorcluster, "TestCase out"=w541:refnum<class "Logging Loopback.lvclass">)  [unwired: 7 in]
            n222 = call "Read Rx Values Until Equal.vi"("expected values"=w510, "error in"=w512, "Rx aliases"=w508, "workspace manager in"=w513) -> ("error out"=w511:errorcluster, "values equal expected"=w509:bool)  [unwired: 5 in, 1 out]
            n223 = call-dynamic "passIf.vi"("error in (no error)"=w511, "pass"=w509, "TestCase in"=w541) -> ("error out"=w484:errorcluster, "TestCase out"=w485:refnum<class "Logging Loopback.lvclass">)  [unwired: 7 in]
          }
          frame Default {
          }
        }
      }
    }
    frame Disabled {
      # "skip test result while test is under development"
      n224 = call <vilib>:"skip.vi"("error in (no error)"=w577, "TestCase in"=w580) -> ("error out"=w579:errorcluster, "TestCase out"=w578:refnum<class "Logging Loopback.lvclass">)  [unwired: 8 in]
    }
  }
  "error out" <- w4
  "TestCase out" <- w2
